vi "Evaluation.vi"(6 "ToEvaluate in":refnum<data-value>, 8 "error in (no error)":errorcluster, 10 "Parents G":dbl, 11 "Tree in":refnum<class "Tree.lvclass">) -> (0 "error out":errorcluster, 1 "H":dbl, 2 "G":dbl, 3 "Tree out":refnum<class "Tree.lvclass">, 4 "ToEvaluate out":refnum<data-value>)   [LabVIEW 2009, in "Tree.lvclass"]
doc: "Abstract method. This is a place holder to override. Use this VI to determine where in the search list OPEN this node belongs. The G value should be the cost of searching to this node. The H value is an approximation of how much farther you need to go to reach your goal node. This only applies to Best First searches."
uses:
  Tree.lvclass
  TreeNode/TreeNode.lvclass
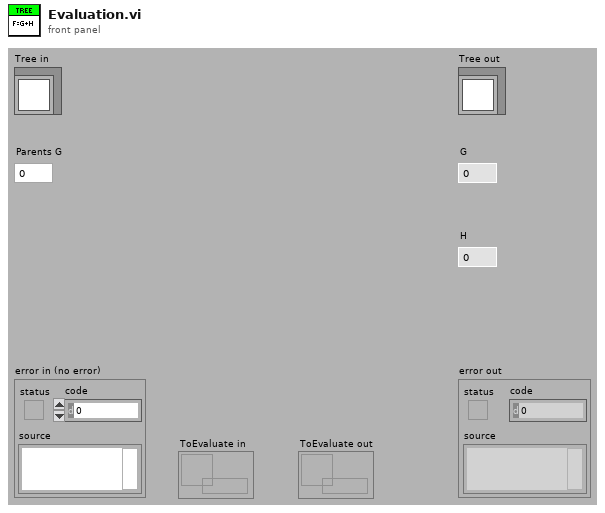
[diagram p1: front panel]
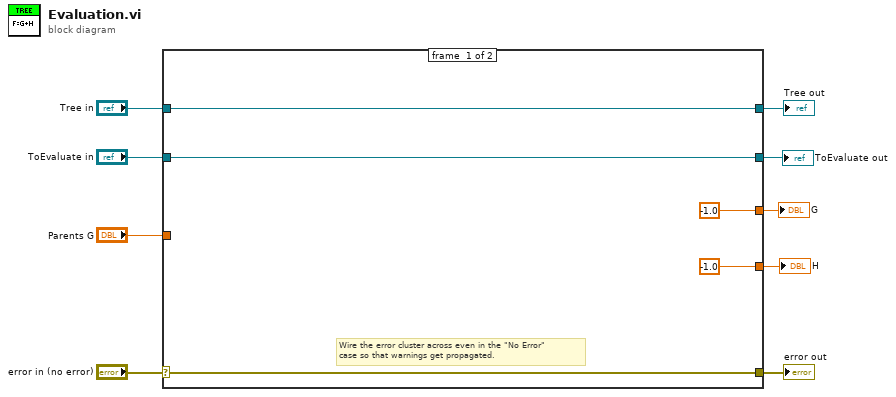
[diagram p0: block diagram]
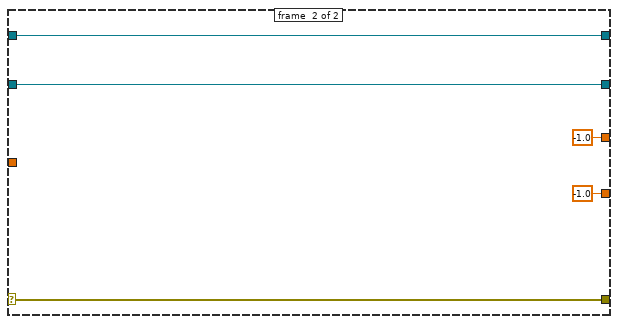
[diagram p2: hidden frame]
diagram:
  n1 = case shown="No Error" "error in (no error)" {
    selector: "error in (no error)" -> [w13 w19]
    tunnel: [w13 w19] -> w8
    tunnel: [w14 w18] -> w6
    tunnel: "Tree in" -> [w14 w18]
    tunnel: "ToEvaluate in" -> [w12 w17]
    tunnel: [w12 w17] -> w4
    tunnel: [-1.0 -1.0] -> w3
    tunnel: [-1.0 -1.0] -> w2
    tunnel: "Parents G" -> [_ _]
    frame #0 {
      # "Wire the error cluster across even in the \"No Error\"\ncase so that warnings get propagated."
    }
    frame #1 {
    }
  }
  "error out" <- w8
  "Tree out" <- w6
  "ToEvaluate out" <- w4
  "G" <- w3
  "H" <- w2
